vi "Walk Structure.vi"(5 "indices":u64[](array[numeric]), 6 "error in (no error)":errorcluster, 8 "variant":variant, 9 "Refnum in":T1) -> (0 "error out":errorcluster, 3 "Refnum out":T1)   [LabVIEW 2019]
uses:
  <vilib>/UPVI/lvhdf5/library.llb/HDF5 Ref.ctl
  <vilib>/Utility/Data Type/Type Definitions/Data Type.ctl
  <vilib>/Utility/miscctls.llb/LVRectTypeDef.ctl
  <vilib>/UPVI/lvhdf5/group.llb/H5G_obj_t.ctl
  <vilib>/UPVI/lvhdf5/dataset.llb/LVH5D Operation.ctl
  <vilib>/UPVI/lvhdf5/group.llb/OpenCreateGroup (String).vi
  <vilib>/UPVI/lvhdf5/utility.llb/Select HDF5 Dialog.vi
  <vilib>/UPVI/lvhdf5/utility.llb/Select HDF5 Dialog (Object Only).vi
  <vilib>/UPVI/lvhdf5/dataset.llb/Simple H5Dwrite (Variant).vi
  <vilib>/UPVI/lvhdf5/dataset.llb/Simple H5Dwrite.xnode
  <vilib>/UPVI/lvhdf5/dataset.llb/H5Dget_space.vi
  <vilib>/UPVI/lvhdf5/dataspace.llb/H5Sselect_hyperslab.vi
  <vilib>/UPVI/lvhdf5/dataset.llb/H5Dwrite (Variant).vi
  <vilib>/UPVI/lvhdf5/dataspace.llb/H5Sclose.vi
  <vilib>/Utility/Data Type/NI_Data Type.lvlib
  <vilib>/UPVI/lvhdf5/file.llb/H5Fclose.vi
  <vilib>/UPVI/lvhdf5/identifier.llb/Not an HDF5 Refnum Constant.vi
  <vilib>/Utility/error.llb/Error Cluster From Error Code.vi
  <vilib>/UPVI/lvhdf5/dataset.llb/OpenCreateReplace Dataset by Element Type.vi
  <vilib>/UPVI/lvhdf5/attribute.llb/private/LVH5AwriteWDTAttrs.vi
  <vilib>/UPVI/lvhdf5/file.llb/OpenCreateReplace HDF5 File.vi
  <vilib>/UPVI/lvhdf5/file.llb/LVH5F Operation.ctl
  <vilib>/UPVI/lvhdf5/utility.llb/Select HDF5 Dialog (File and Object).vi
panel:
  out "Fieldnames":string[](array[string])
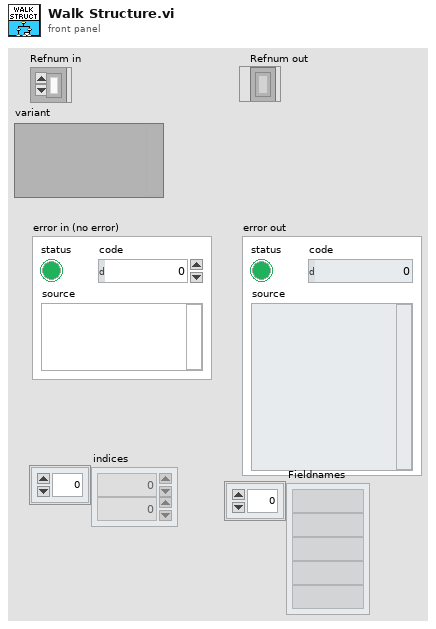
[diagram p1: front panel]
types:
  T1 = typedef "HDF5 Ref.ctl" = refnum<k1>
  T2 = typedef "NI_Data Type.lvlib/Data Type.ctl" = enum8{"Invalid Type", "Void", "I8", "I16", "I32", "I64", "U8", "U16", "U32", "U64", "Single Float", "Double Float", "Extended Float", "Single Complex", "Double Complex", "Extended Complex", "Enum U8", "Enum U16", "Enum U32", "Enum U64", "Single Float With Unit", "Double Float With Unit", "Extended Float With Unit", "Single Complex with Unit", "Double Complex with Unit", "Extended Complex with Unit", "Boolean", "String", "Path", "Picture", "Tag", "Array", "Cluster", "Variant", "LV Variant", "Waveform", "Timestamp", "Digital Waveform", "Digital Data", "ExpressData", "Refnum", "External Data", "VI", "Poly VI", "LabVIEW Class Instance", "Fixed Point", "Set Collection", "Map Collection"}
  T3 = typedef "LVRectTypeDef.ctl" = cluster{"Left":i16, "Top":i16, "Right":i16, "Bottom":i16}
  T4 = cluster{"Behavior":enum32{"Invalid", "Default", "Floating", "Floating/Auto-Hide", "Modal"}, "Position":T3, "Center":bool, "Title":string}
  T5 = typedef "LVH5F Operation.ctl" = enum16{"open", "open or create", "create or replace", "create or replace (with confirmation)", "create", "open (read only)"}
  T6 = typedef "LVH5D Operation.ctl" = enum16{"open", "replace", "create", "open or create", "create or replace", "create or replace with confirmation"}
  T7 = typedef "H5G_obj_t.ctl" = i32
  T8 = cluster{"Object Types (any)":T7[], "Object Pattern":string}
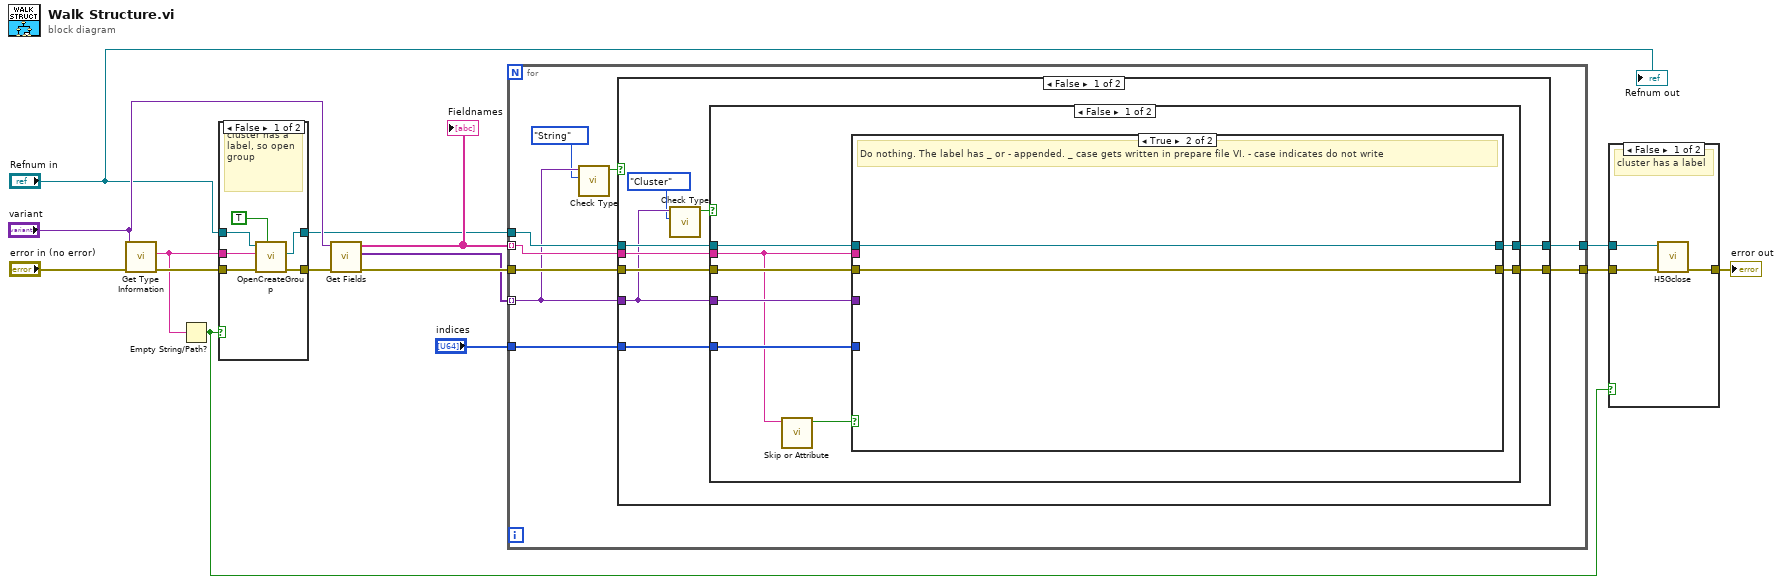
[diagram p0: block diagram]
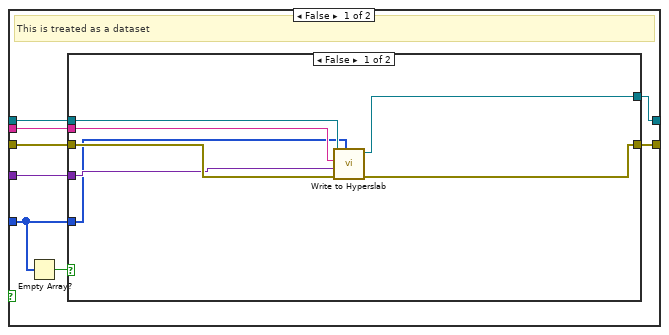
[diagram p4: hidden frame]
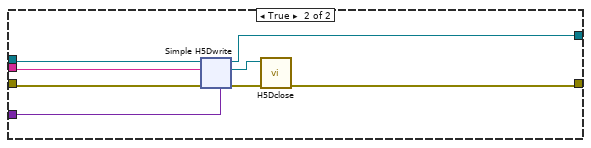
[diagram p5: hidden frame]
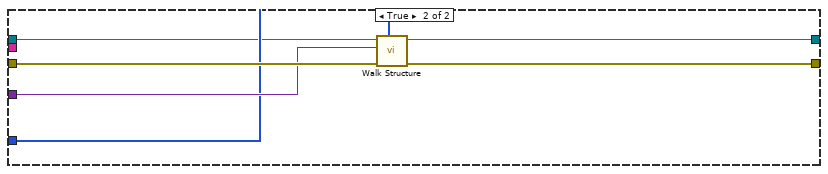
[diagram p6: hidden frame]
diagram:
  n1 = call <vilib>:"Get Type Information.vi"("error in (no error)"="error in (no error)", "variant"="variant") -> ("error out"=w11:errorcluster, "name"=w5:string)  [unwired: 5 in, 3 out]
  n2 = Empty String/Path?(string/path=w5) -> (empty?=w2:bool)
  n3 = case shown="False" w2 {
    tunnel: w11 -> [w21 w23]
    tunnel: w5 -> [w20 _]
    tunnel: [w19 w23] -> w9
    tunnel: [w16 w22] -> w4
    tunnel: "Refnum in" -> [w18 w22]
    frame False {
      # "cluster has a label, so open group"
      n4 = call-poly <vilib>:"OpenCreateGroup.vi"("Create if not found (F)"=TRUE, "error in (no error)"=w21, "Group"=w20, "HDF5 Ref"=w18) -> ("error out"=w19:errorcluster, "HDF5 Group Ref"=w16:T1)  [unwired: 5 in, 1 out]
    }
    frame True {
      # "cluster has no label"
    }
  }
  n5 = call "Get Fields.vi"("error in (no error)"=w9, "variant"="variant") -> ("error out"=w15:errorcluster, "element variant array"=w13:variant[], "Fieldnames"=w14:string[])  [unwired: 5 in, 2 out]
  "Fieldnames" <- w14
  n6 = for {
    tunnel: w4 -> [w32]
    tunnel: [w31] -> w1
    tunnel: [w30] -> w7
    tunnel: w14 -> [w29] mode=indexing
    tunnel: w15 -> [w28]
    tunnel: w13 -> [w26] mode=indexing
    tunnel: "indices" -> [w27]
    n7 = call "Check Type.vi"("type"=Data_Type."String", "variant"=w26) -> ("is type"=w25:bool)  [unwired: 8 in, 1 out]
    n8 = case shown="False" w25 {
      tunnel: w32 -> [w41 w284]
      tunnel: [w40 w284] -> w31
      tunnel: [w39 w283] -> w30
      tunnel: w29 -> [w37 _]
      tunnel: w28 -> [w36 w283]
      tunnel: w26 -> [w35 _]
      tunnel: w27 -> [w34 _]
      frame False {
        n9 = call "Check Type.vi"("type"=Data_Type."Cluster", "variant"=w35) -> ("is type"=w38:bool)  [unwired: 8 in, 1 out]
        n10 = case shown="False" w38 {
          tunnel: w41 -> [w49 w278]
          tunnel: w37 -> [w43 _]
          tunnel: [w46 w277] -> w40
          tunnel: [w45 w281] -> w39
          tunnel: w36 -> [w48 w282]
          tunnel: w35 -> [w47 w280]
          tunnel: w34 -> [w44 w279]
          frame False {
            n11 = call "Skip or Attribute.vi"("Label.Text"=w43) -> ("Checkbox"=w42:bool)  [unwired: 10 in]
            n12 = case shown="True" w42 {
              tunnel: w49 -> [w57 w276]
              tunnel: w48 -> [w56 w275]
              tunnel: w43 -> [w55 _]
              tunnel: w47 -> [w54 _]
              tunnel: [w53 w276] -> w46
              tunnel: [w52 w275] -> w45
              tunnel: w44 -> [w51 _]
              frame False {
                # "This is treated as a dataset"
                n13 = Empty Array?(array=w51) -> (empty?=w50:bool)
                n14 = case shown="False" w50 {
                  tunnel: w57 -> [w64 w72]
                  tunnel: w56 -> [w63 w69]
                  tunnel: w55 -> [w62 w70]
                  tunnel: w54 -> [w61 w71]
                  tunnel: [w60 w67] -> w53
                  tunnel: [w59 w65] -> w52
                  tunnel: w51 -> [w58 _]
                  frame False {
                    n15 = call "Write to Hyperslab.vi"("indices"=w58, "error in (no error)"=w63, "Variant"=w61, "Label.Text"=w62, "Refnum in"=w64) -> ("error out"=w59:errorcluster, "Refnum out"=w60:T1)  [unwired: 5 in]
                  }
                  frame True {
                    n16 = xnode "Simple H5Dwrite"("Dataset Path"=w70, "error in (no error)"=w69, "HDF5 Path or Ref"=w72, "Data"=w71) -> ("HDF5 Dataset Ref out"=w66:T1, "HDF5 Ref out"=w67:T1, "error out"=w68:errorcluster)  [unwired: 4 in]
                    n17 = call <vilib>:"H5Dclose.vi"("error in (no error)"=w68, "HDF5 Dataset Ref"=w66) -> ("error out"=w65:errorcluster)  [unwired: 7 in]
                  }
                }
              }
              frame True {
                # "Do nothing. The label has _ or - appended. _ case gets written in prepare file VI. - case indicates do not write"
              }
            }
          }
          frame True {
            n18 = call "Walk Structure.vi"("indices"=w279, "error in (no error)"=w282, "variant"=w280, "Refnum in"=w278) -> ("error out"=w281:errorcluster, "Refnum out"=w277:T1)  [unwired: 4 in]
          }
        }
      }
      frame True {
        # "#TODO Can't write strings"
      }
    }
  }
  n19 = case shown="False" w2 {
    tunnel: w7 -> [w287 w288]
    tunnel: [w286 w288] -> w6
    tunnel: w1 -> [w285 _]
    frame False {
      # "cluster has a label"
      n20 = call <vilib>:"H5Gclose.vi"("error in (no error)"=w287, "HDF5 Group Ref"=w285) -> ("error out"=w286:errorcluster)  [unwired: 7 in]
    }
    frame True {
      # "cluster has no label"
    }
  }
  "error out" <- w6
  "Refnum out" <- "Refnum in"
